vi "Default Settings.vi"() -> (3 "Default Settings":T1)   [LabVIEW 2019, in "Settings Editor.lvlib"]
doc: "_____\nBased on DQMH Project Template 6.0.0.91."
uses:
  Settings Editor.lvlib
  Settings--cluster.ctl
  CML Shared/Signal Type--enum.ctl
  CML Shared/Calibration Values--cluster.ctl
  <vilib>/Utility/sysdir.llb/System Directory Type.ctl
  CML Shared/CML Shared.lvlib
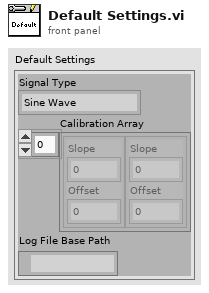
[diagram p1: front panel]
types:
  T1 = typedef "Settings Editor.lvlib/Settings--cluster.ctl" = cluster{"Signal Type":T2, "Calibration Array":T3[], "Log File Base Path":path}
  T2 = typedef "CML Shared.lvlib/Signal Type--enum.ctl" = enum16{"Sine Wave", "Square with Noise"}
  T3 = typedef "CML Shared.lvlib/Calibration Values--cluster.ctl" = cluster{"Slope":dbl, "Offset":dbl}
  T4 = typedef "System Directory Type.ctl" = i32
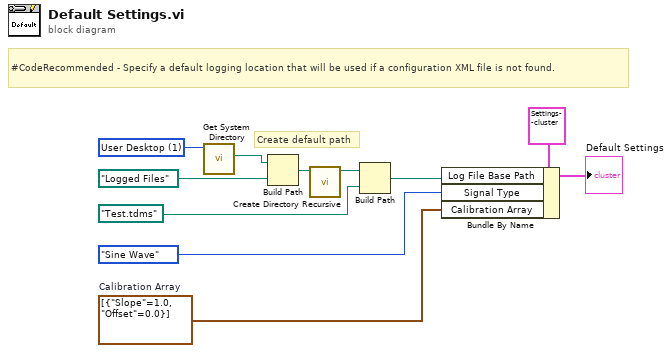
[diagram p0: block diagram]
diagram:
  w3 = T3[] [{"Slope"=1.0, "Offset"=0.0}]  # Calibration Array
  w11 = T4 1 items=["User Home"=0, "User Desktop"=1, "User Documents"=2, "User Application Data"=3, "User Preferences"=4, "User Temporary"=5, "Public Documents"=6, "Public Application Data"=7, "Public Preferences"=8, "Public Cache"=13, "System Core Libraries"=9, "System Installed Libraries"=10, "Application Files"=11, "Boot Volume Root"=12] ("system directory type")
  # "#CodeRecommended - Specify a default logging location that will be used if a configuration XML file is not found."
  # "Create default path"
  n1 = call <vilib>:"Get System Directory.vi"("system directory type"=w11) -> ("system directory"=w10:path)  [unwired: 10 in]
  n2 = Build Path(base path=w10, name or relative path=path "Logged Files") -> (appended path=w9:path)
  n3 = call <vilib>:"Create Directory Recursive.vi"("directory"=w9) -> ("directory copy"=w8:path)  [unwired: 4 in, 2 out]
  n4 = Build Path(base path=w8, name or relative path=path "Test.tdms") -> (appended path=w5:path)
  n5 = Bundle By Name(cluster=T1 {"Signal Type"=enum."Sine Wave", "Calibration Array"=[{"Slope"=1.0, "Offset"=0.0}], "Log File Base Path"=path ""} ("Default Settings"), "Log File Base Path"=w5, "Signal Type"=Signal_Type--enum."Sine Wave", "Calibration Array"=w3) -> (→"Default Settings":T1)
